vi "Goto.vi"(6 "Home?":bool, 7 "Speed":i32, 8 "error in (no error)":errorcluster, 9 "channel":i32(ring)=1 items=["Channel1"=1, "Channel2"=2, "Channel3"=3, "Channel4"=4], 10 "New Position":i32, 11 "TranslationStage in":refnum<class "KIM101.lvclass">) -> (0 "error out":errorcluster, 3 "TranslationStage out":refnum<class "KIM101.lvclass">)   [LabVIEW 2023, in "KIM101.lvlib" / "KIM101.lvclass"]
uses:
  KIM101.lvclass
  UIs/TranslationStage_UI/TranslationStage_UI/StageMoveDone_For_UI.ctl
  KIM101.lvclass/KIM101.ctl
  <vilib>/ActorFramework/Actor/Actor.lvclass/Actor.ctl
  Interfaces/AbstractInstrumentClasses/TranslationStages_LV/TranslationStagesComm Messages/StageMoveDone Msg/StageMoveDone Msg.lvclass/StageMoveDone Msg.ctl
  <vilib>/ActorFramework/Message Enqueuer/Message Enqueuer.lvclass/Message Enqueuer.ctl
  <vilib>/ActorFramework/Message Enqueuer/Enqueue.vi
  Interfaces/AbstractInstrumentClasses/TranslationStages_LV/TranslationStagesComm Messages/StageMoveDone Msg/StageMoveDone Msg.lvclass
  C:/Users/quantum/Documents/LVDAQ/UIs/TranslationStage_UI/Thorlabs.MotionControl.KCube.InertialMotorCLI.dll
  UIs/TranslationStage_UI/Thorlabs.MotionControl.KCube.InertialMotorCLI.dll
  <vilib>/ActorFramework/Message Priority Queue/Priority Enqueue.vi
  <vilib>/ActorFramework/Actor/Actor.lvclass
  typedefs/typedefs.lvlib
panel:
  in  "Positions":T1={"CH1 Pos"=0.0, "CH2 Pos"=0.0, "CH3 Pos"=0.0, "CH4 Pos"=0.0, "Home?"=TRUE}
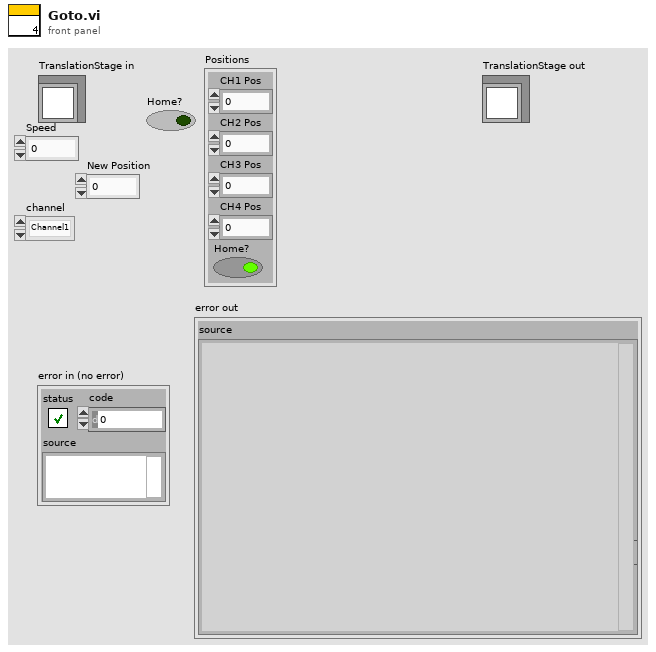
[diagram p1: front panel]
types:
  T1 = typedef "typedefs.lvlib/StageMoveDone_For_UI.ctl" = cluster{"CH1 Pos":dbl, "CH2 Pos":dbl, "CH3 Pos":dbl, "CH4 Pos":dbl, "Home?":bool}
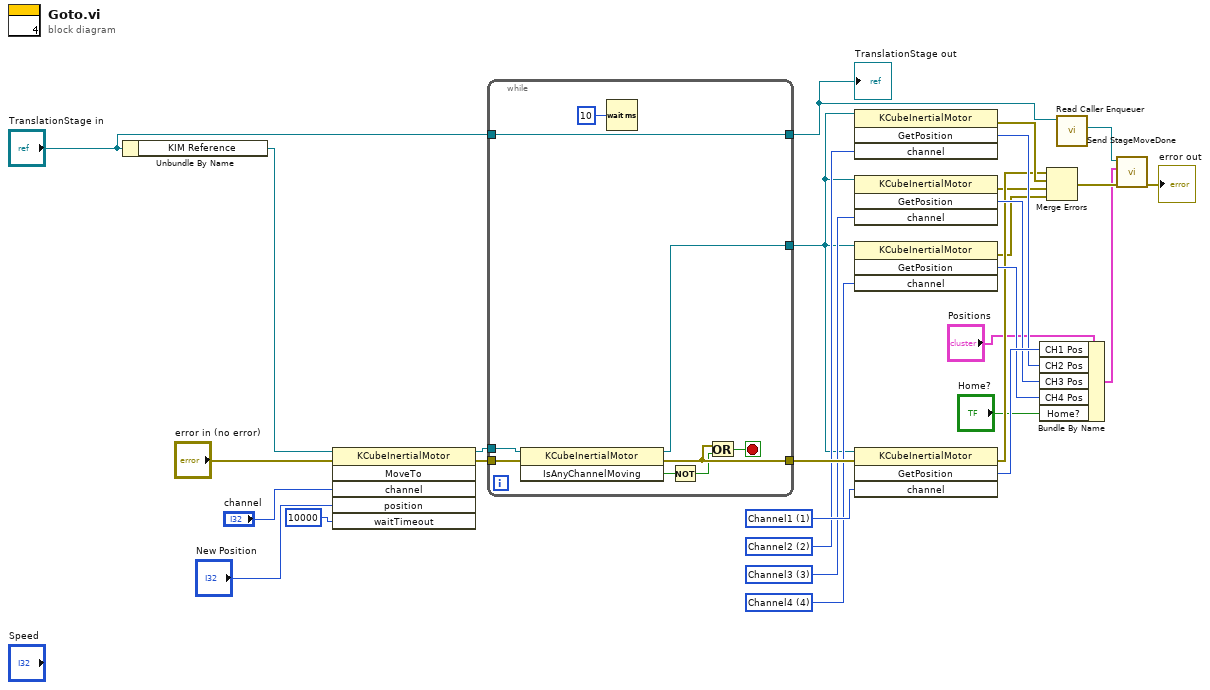
[diagram p0: block diagram]
diagram:
  w24 = 4 items=["Channel1"=1, "Channel2"=2, "Channel3"=3, "Channel4"=4] ("channel")
  w25 = 3 items=["Channel1"=1, "Channel2"=2, "Channel3"=3, "Channel4"=4] ("channel")
  w26 = 2 items=["Channel1"=1, "Channel2"=2, "Channel3"=3, "Channel4"=4] ("channel")
  w27 = 1 items=["Channel1"=1, "Channel2"=2, "Channel3"=3, "Channel4"=4] ("channel")
  n1 = Unbundle By Name("TranslationStage in") -> ("KIM Reference"=w7:refnum<k24>)
  n2 = invoke class="KCubeInertialMotor" method="MoveTo"(reference=w7, error in="error in (no error)", "channel"="channel", "position"="New Position", "waitTimeout"=10000) -> (reference out=w4:refnum<k24>, error out=w5:errorcluster)  [unwired: 1 in, 4 out]
  n3 = while {
    tunnel: [w35] -> w28
    tunnel: [w38] -> w11
    tunnel: "TranslationStage in" -> [w38]
    tunnel: [w32] -> w14
    tunnel: w5 -> [w31]
    tunnel: w4 -> [w30]
    stop <- w34 stop-if-true
    n4 = invoke class="KCubeInertialMotor" method="IsAnyChannelMoving"(reference=w30, error in=w31) -> (reference out=w32:refnum<k24>, error out=w35:errorcluster, "IsAnyChannelMoving"=w36:bool)  [unwired: 1 in]
    n5 = Wait (ms)(milliseconds to wait=u32 10) -> ()  [unwired: 1 out]
    n6 = Not(x=w36) -> (.not. x?=w33:bool)
    n7 = Or(x=w35, y=w33) -> (x .or. y?=w34:bool)
  }
  "TranslationStage out" <- w11
  n8 = invoke class="KCubeInertialMotor" method="GetPosition"(reference=w14, "channel"=w26) -> (error out=w19:errorcluster, "GetPosition"=w22:i32)  [unwired: 2 in, 2 out]
  n9 = invoke class="KCubeInertialMotor" method="GetPosition"(reference=w14, "channel"=w25) -> (error out=w16:errorcluster, "GetPosition"=w21:i32)  [unwired: 2 in, 2 out]
  n10 = invoke class="KCubeInertialMotor" method="GetPosition"(reference=w14, "channel"=w24) -> (error out=w15:errorcluster, "GetPosition"=w20:i32)  [unwired: 2 in, 2 out]
  n11 = invoke class="KCubeInertialMotor" method="GetPosition"(reference=w14, error in=w28, "channel"=w27) -> (error out=w18:errorcluster, "GetPosition"=w23:i32)  [unwired: 1 in, 2 out]
  n12 = Bundle By Name(cluster="Positions", "CH1 Pos"=w23, "CH2 Pos"=w22, "CH3 Pos"=w21, "CH4 Pos"=w20, "Home?"="Home?") -> (w13:T1)
  n13 = Merge Errors(w18, w19, w16, w15) -> (w17:errorcluster)
  n14 = call <vilib>:"Read Caller Enqueuer.vi"("Actor"=w11) -> ("Caller Enqueuer"=w29:refnum<class "Message Enqueuer.lvclass">)  [unwired: 10 in]
  n15 = call "Send StageMoveDone.vi"("error in (no error)"=w17, "Positions"=w13, "Message Enqueuer"=w29) -> ("error out"=→"error out":errorcluster)  [unwired: 7 in, 1 out]
